vi "Max Search.vi"() -> ()   [LabVIEW 2025]
panel:
  out "Iteration Count":i32
  out "Random Number":dbl
  out "Max":dbl
  in  "Number of Iterations":i32
  # "ME 235: Design of Microprocessor Based Mechanical Systems"
  # "Lab 1 - Max Search"
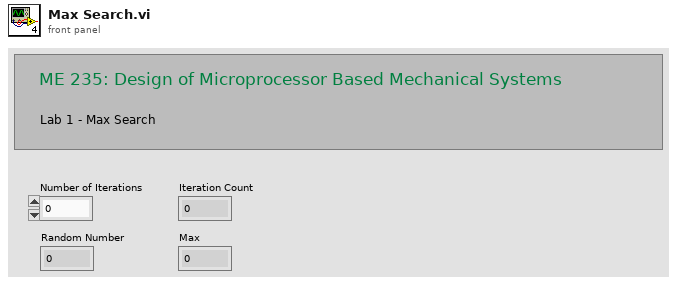
[diagram p1: front panel]
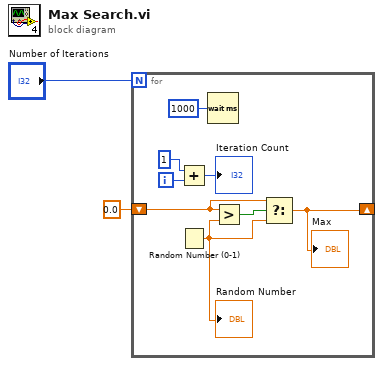
[diagram p0: block diagram]
diagram:
  n1 = for {
    N: "Number of Iterations" -> [_]
    shift-right: [w4] -> _
    shift-left: 0.0 -> [w5]
    i -> [w9]
    n2 = Add(x=1, y=w9) -> (x+y=→"Iteration Count":i32)
    n3 = Random Number (0-1)() -> (number: 0 to 1=w7:dbl)
    "Random Number" <- w7
    n4 = Wait (ms)(milliseconds to wait=u32 1000) -> ()  [unwired: 1 out]
    n5 = Greater?(x=w5, y=w7) -> (0:w6:bool)
    n6 = Select(t=w5, s=w6, f=w7) -> (s? t:f=w4:dbl)
    "Max" <- w4
  }
